vi "자판기.vi"() -> ()   [LabVIEW 2020]
panel:
  in  "정지":bool
  in  "거스름돈 반환":bool
  out "배출 상품명":string
  out "현재 잔액":dbl
  out "웰치스 LED":bool
  in  "웰치스":bool
  out "콜라 LED":bool
  in  "콜라":bool
  out "환타 LED":bool
  in  "환타":bool
  out "사이다 LED":bool
  in  "1000원":bool
  in  "500원":bool
  in  "100원":bool
  in  "10원":bool
  in  "50 원":bool
  in  "사이다":bool
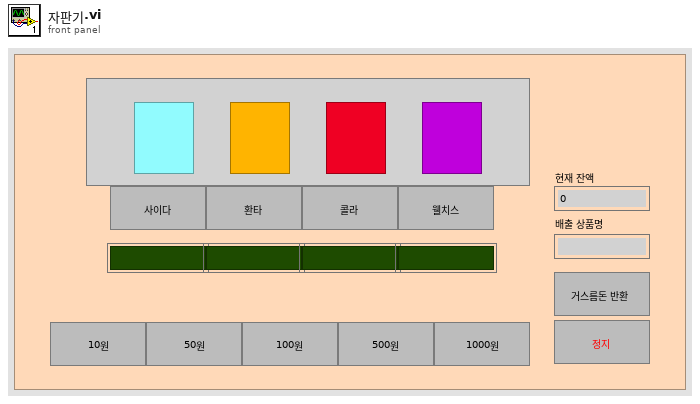
[diagram p1: front panel]
types:
  T1 = typedef "컨트롤 1.ctl" = enum16{"초기화", "대기", "10원", "50원", "100원", "500원", "1000원", "디스플레이 업데이트", "사이다", "콜라", "환타", "웰치스", "거스름돈 반환", "종료"}
  T2 = cluster{"배출 상품명":string, "현재 잔액":dbl, "웰치스 LED":bool, "콜라 LED":bool, "환타 LED":bool, "사이다 LED":bool}
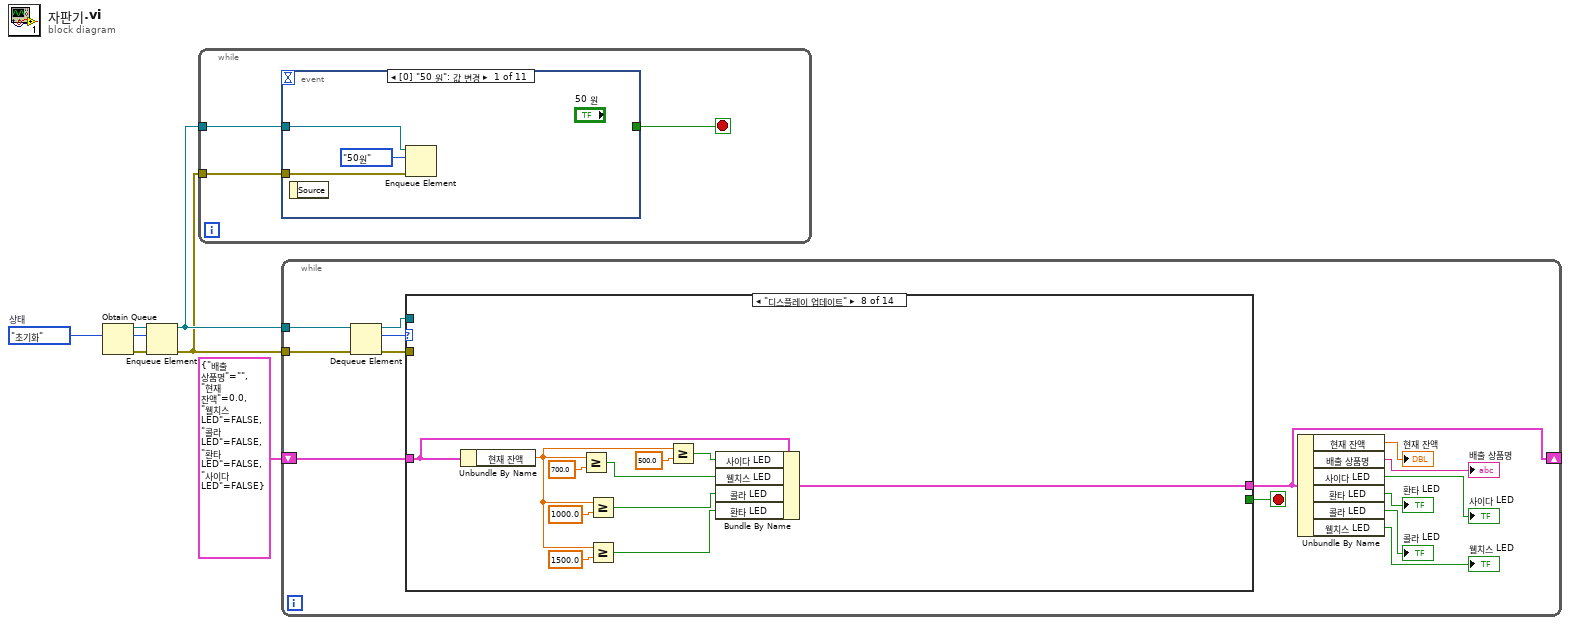
[diagram p0: block diagram]
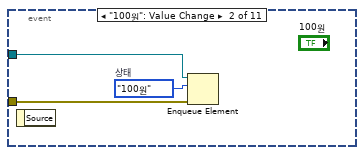
[diagram p2: hidden frame]
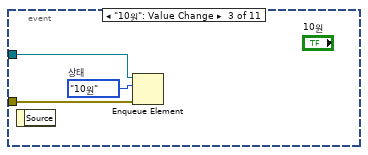
[diagram p3: hidden frame]
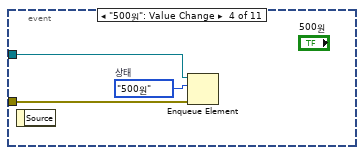
[diagram p4: hidden frame]
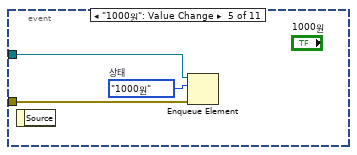
[diagram p5: hidden frame]
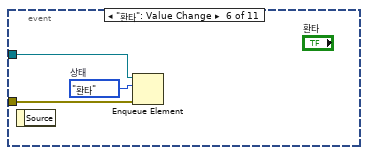
[diagram p6: hidden frame]
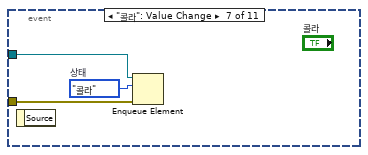
[diagram p7: hidden frame]
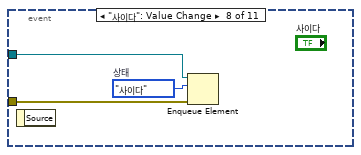
[diagram p8: hidden frame]
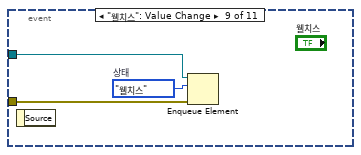
[diagram p9: hidden frame]
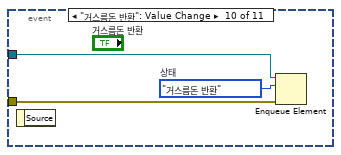
[diagram p10: hidden frame]
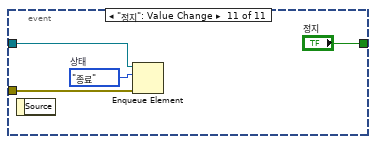
[diagram p11: hidden frame]
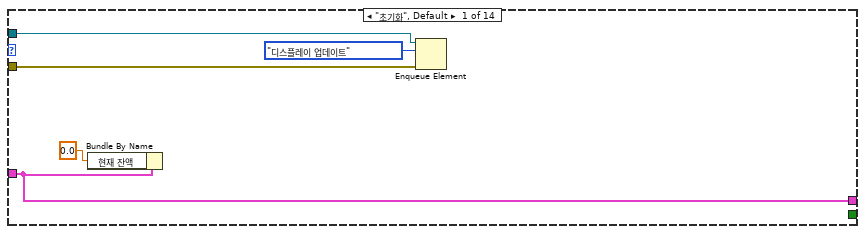
[diagram p12: hidden frame]
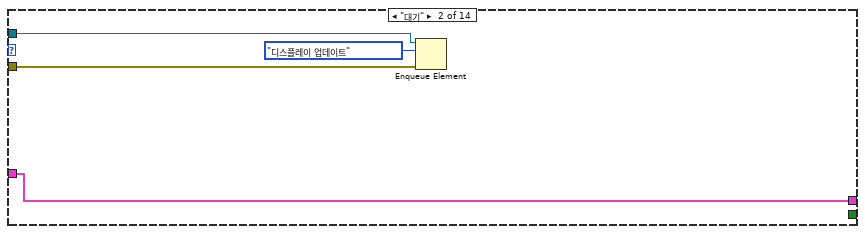
[diagram p13: hidden frame]
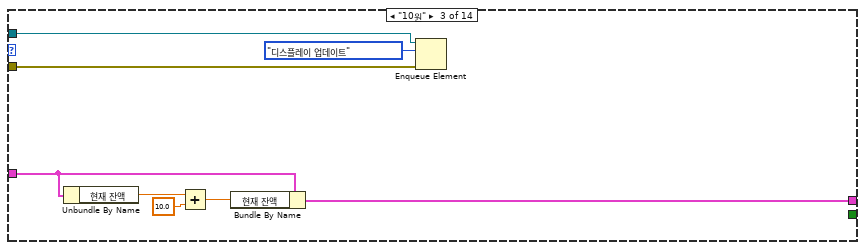
[diagram p14: hidden frame]
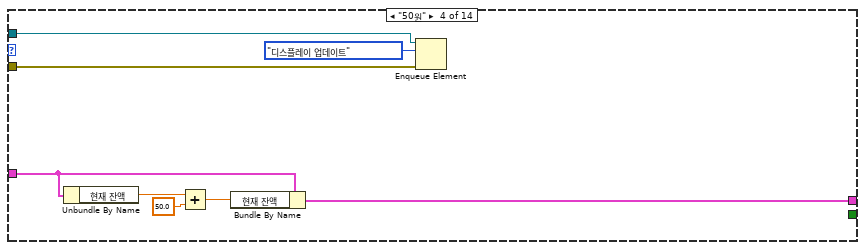
[diagram p15: hidden frame]
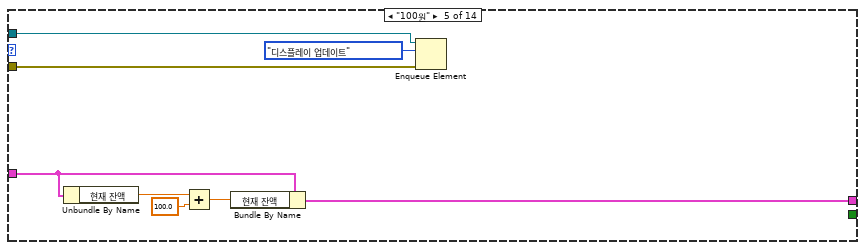
[diagram p16: hidden frame]
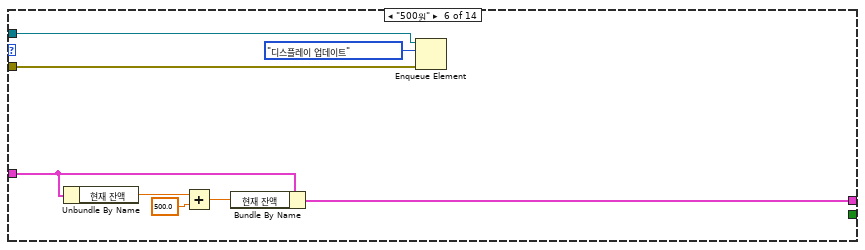
[diagram p17: hidden frame]
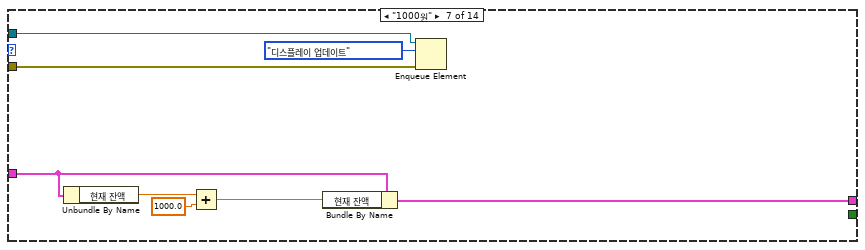
[diagram p18: hidden frame]
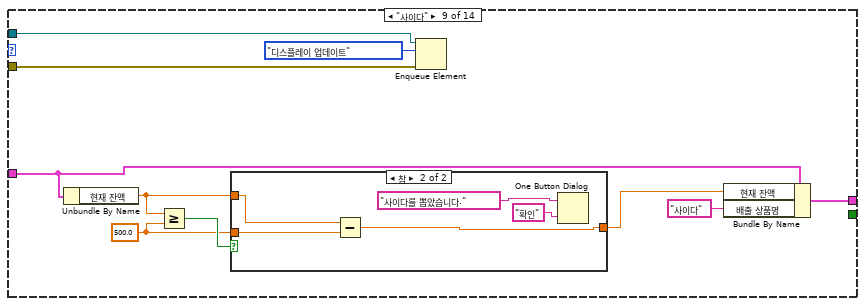
[diagram p19: hidden frame]
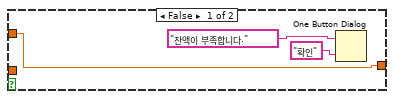
[diagram p20: hidden frame]
diagram:
  w4 = 컨트롤_1."초기화"  # 상태
  n1 = Obtain Queue(element data type=w4) -> (queue out=w5:refnum<queue>, error out=w3:errorcluster)  [unwired: 4 in, 1 out]
  n2 = Enqueue Element(queue=w5, element=w4, error in (no error)=w3) -> (queue out=w2:refnum<queue>, error out=w1:errorcluster)  [unwired: 1 in, 1 out]
  n3 = while {
    tunnel: w2 -> [w9]
    tunnel: w1 -> [w8]
    stop <- w7 stop-if-true
    n4 = event shown="[0] \"50 원\": 값 변경" {
      selector: _ -> [_ _ _ _ _ _ _ _ _ _ _]
      dyn-events: _ -> [_ _ _ _ _ _ _ _ _ _ _]
      timeout: _ -> [_ _ _ _ _ _ _ _ _ _ _]
      tunnel: w9 -> [w12 w15 w18 w21 w24 w27 w30 w33 w36 w39 w43]
      tunnel: w8 -> [w11 w14 w17 w20 w23 w26 w29 w32 w35 w38 w42]
      tunnel: [_ _ _ _ _ _ _ _ _ _ "정지"] -> w7
      event "50 원": Value Change {
        n5 = event-data() -> ()  [unwired: 1 in, 1 out]
        n6 = Enqueue Element(queue=w12, element=컨트롤_1."50원" ("원소"), error in (no error)=w11) -> ()  [unwired: 1 in, 3 out]
      }
      event "100원": Value Change {
        w13 = 컨트롤_1."100원"  # 상태
        n7 = event-data() -> ()  [unwired: 1 in, 1 out]
        n8 = Enqueue Element(queue=w15, element=w13, error in (no error)=w14) -> ()  [unwired: 1 in, 3 out]
      }
      event "10원": Value Change {
        w16 = 컨트롤_1."10원"  # 상태
        n9 = event-data() -> ()  [unwired: 1 in, 1 out]
        n10 = Enqueue Element(queue=w18, element=w16, error in (no error)=w17) -> ()  [unwired: 1 in, 3 out]
      }
      event "500원": Value Change {
        w19 = 컨트롤_1."500원"  # 상태
        n11 = event-data() -> ()  [unwired: 1 in, 1 out]
        n12 = Enqueue Element(queue=w21, element=w19, error in (no error)=w20) -> ()  [unwired: 1 in, 3 out]
      }
      event "1000원": Value Change {
        w22 = 컨트롤_1."1000원"  # 상태
        n13 = event-data() -> ()  [unwired: 1 in, 1 out]
        n14 = Enqueue Element(queue=w24, element=w22, error in (no error)=w23) -> ()  [unwired: 1 in, 3 out]
      }
      event "환타": Value Change {
        w25 = 컨트롤_1."환타"  # 상태
        n15 = event-data() -> ()  [unwired: 1 in, 1 out]
        n16 = Enqueue Element(queue=w27, element=w25, error in (no error)=w26) -> ()  [unwired: 1 in, 3 out]
      }
      event "콜라": Value Change {
        w28 = 컨트롤_1."콜라"  # 상태
        n17 = event-data() -> ()  [unwired: 1 in, 1 out]
        n18 = Enqueue Element(queue=w30, element=w28, error in (no error)=w29) -> ()  [unwired: 1 in, 3 out]
      }
      event "사이다": Value Change {
        w31 = 컨트롤_1."사이다"  # 상태
        n19 = event-data() -> ()  [unwired: 1 in, 1 out]
        n20 = Enqueue Element(queue=w33, element=w31, error in (no error)=w32) -> ()  [unwired: 1 in, 3 out]
      }
      event "웰치스": Value Change {
        w34 = 컨트롤_1."웰치스"  # 상태
        n21 = event-data() -> ()  [unwired: 1 in, 1 out]
        n22 = Enqueue Element(queue=w36, element=w34, error in (no error)=w35) -> ()  [unwired: 1 in, 3 out]
      }
      event "거스름돈 반환": Value Change {
        w37 = 컨트롤_1."거스름돈 반환"  # 상태
        n23 = event-data() -> ()  [unwired: 1 in, 1 out]
        n24 = Enqueue Element(queue=w39, element=w37, error in (no error)=w38) -> ()  [unwired: 1 in, 3 out]
      }
      event "정지": Value Change {
        w41 = 컨트롤_1."종료"  # 상태
        n25 = event-data() -> ()  [unwired: 1 in, 1 out]
        n26 = Enqueue Element(queue=w43, element=w41, error in (no error)=w42) -> ()  [unwired: 1 in, 3 out]
      }
    }
  }
  n27 = while {
    shift-right: [w56] -> _
    shift-left: T2 {"배출 상품명"="", "현재 잔액"=0.0, "웰치스 LED"=FALSE, "콜라 LED"=FALSE, "환타 LED"=FALSE, "사이다 LED"=FALSE} -> [w57]
    tunnel: w2 -> [w49]
    tunnel: w1 -> [w48]
    stop <- w44 stop-if-true
    n28 = Dequeue Element(queue=w49, error in (no error)=w48) -> (queue out=w46:refnum<queue>, element=w47:T1, error out=w45:errorcluster)  [unwired: 1 in, 1 out]
    n29 = case shown="\"디스플레이 업데이트\"" w47 {
      tunnel: w57 -> [w58 w63 w68 w80 w88 w92 w100 w113 w124 w141 w158 w177 w196 w202]
      tunnel: [w58 w63 w67 w78 w86 w91 w99 w107 w123 w140 w159 w174 w199 w202] -> w56
      tunnel: w46 -> [w61 w65 w70 w77 w85 w94 w102 _ w121 w139 w157 w176 w198 w204]
      tunnel: w45 -> [w60 w64 w69 w75 w83 w93 w101 _ w120 w138 w156 w175 w197 w203]
      tunnel: [_ _ _ _ _ _ _ _ _ _ _ _ _ TRUE] -> w44
      frame "초기화", Default {
        n30 = Bundle By Name(cluster=w58, "현재 잔액"=0.0) -> ()  [unwired: 1 out]
        n31 = Enqueue Element(queue=w61, element=컨트롤_1."디스플레이 업데이트" ("원소"), error in (no error)=w60) -> ()  [unwired: 1 in, 3 out]
      }
      frame "대기" {
        n32 = Enqueue Element(queue=w65, element=컨트롤_1."디스플레이 업데이트" ("원소"), error in (no error)=w64) -> ()  [unwired: 1 in, 3 out]
      }
      frame "10원" {
        n33 = Unbundle By Name(w68) -> ("현재 잔액"=w74:dbl)
        n34 = Add(x=w74, y=10.0) -> (x+y=w72:dbl)
        n35 = Bundle By Name(cluster=w68, "현재 잔액"=w72) -> (w67:T2)
        n36 = Enqueue Element(queue=w70, element=컨트롤_1."디스플레이 업데이트" ("원소"), error in (no error)=w69) -> ()  [unwired: 1 in, 3 out]
      }
      frame "50원" {
        n37 = Unbundle By Name(w80) -> ("현재 잔액"=w82:dbl)
        n38 = Add(x=w82, y=50.0) -> (x+y=w79:dbl)
        n39 = Bundle By Name(cluster=w80, "현재 잔액"=w79) -> (w78:T2)
        n40 = Enqueue Element(queue=w77, element=컨트롤_1."디스플레이 업데이트" ("원소"), error in (no error)=w75) -> ()  [unwired: 1 in, 3 out]
      }
      frame "100원" {
        n41 = Unbundle By Name(w88) -> ("현재 잔액"=w90:dbl)
        n42 = Add(x=w90, y=100.0) -> (x+y=w87:dbl)
        n43 = Bundle By Name(cluster=w88, "현재 잔액"=w87) -> (w86:T2)
        n44 = Enqueue Element(queue=w85, element=컨트롤_1."디스플레이 업데이트" ("원소"), error in (no error)=w83) -> ()  [unwired: 1 in, 3 out]
      }
      frame "500원" {
        n45 = Unbundle By Name(w92) -> ("현재 잔액"=w97:dbl)
        n46 = Add(x=w97, y=500.0) -> (x+y=w98:dbl)
        n47 = Bundle By Name(cluster=w92, "현재 잔액"=w98) -> (w91:T2)
        n48 = Enqueue Element(queue=w94, element=컨트롤_1."디스플레이 업데이트" ("원소"), error in (no error)=w93) -> ()  [unwired: 1 in, 3 out]
      }
      frame "1000원" {
        n49 = Unbundle By Name(w100) -> ("현재 잔액"=w105:dbl)
        n50 = Add(x=w105, y=1000.0) -> (x+y=w106:dbl)
        n51 = Bundle By Name(cluster=w100, "현재 잔액"=w106) -> (w99:T2)
        n52 = Enqueue Element(queue=w102, element=컨트롤_1."디스플레이 업데이트" ("원소"), error in (no error)=w101) -> ()  [unwired: 1 in, 3 out]
      }
      frame "디스플레이 업데이트" {
        n53 = Unbundle By Name(w113) -> ("현재 잔액"=w112:dbl)
        n54 = Greater Or Equal?(x=w112, y=700.0) -> (x >= y?=w110:bool)
        n55 = Greater Or Equal?(x=w112, y=1000.0) -> (x >= y?=w109:bool)
        n56 = Greater Or Equal?(x=w112, y=1500.0) -> (x >= y?=w108:bool)
        n57 = Greater Or Equal?(x=w112, y=500.0) -> (x >= y?=w111:bool)
        n58 = Bundle By Name(cluster=w113, "사이다 LED"=w111, "웰치스 LED"=w110, "콜라 LED"=w109, "환타 LED"=w108) -> (w107:T2)
      }
      frame "사이다" {
        w119 = 500.0 ("y")
        n59 = Unbundle By Name(w124) -> ("현재 잔액"=w126:dbl)
        n60 = Greater Or Equal?(x=w126, y=w119) -> (x >= y?=w127:bool)
        n61 = case shown="참" w127 {
          tunnel: w126 -> [w130 w135]
          tunnel: [w130 w134] -> w125
          tunnel: w119 -> [_ w131]
          frame False {
            n62 = One Button Dialog(message="잔액이 부족합니다." ("메시지"), button name ("OK")="확인" ("버튼 이름(\"확인\")")) -> ()  [unwired: 1 out]
          }
          frame True {
            n63 = Subtract(x=w135, y=w131) -> (x-y=w134:dbl)
            n64 = One Button Dialog(message="사이다를 뽑았습니다." ("메시지"), button name ("OK")="확인" ("버튼 이름(\"확인\")")) -> ()  [unwired: 1 out]
          }
        }
        n65 = Enqueue Element(queue=w121, element=컨트롤_1."디스플레이 업데이트" ("원소"), error in (no error)=w120) -> ()  [unwired: 1 in, 3 out]
        n66 = Bundle By Name(cluster=w124, "현재 잔액"=w125, "배출 상품명"="사이다") -> (w123:T2)
      }
      frame "콜라" {
        w137 = 1000.0 ("y")
        n67 = Unbundle By Name(w141) -> ("현재 잔액"=w144:dbl)
        n68 = Greater Or Equal?(x=w144, y=w137) -> (x >= y?=w145:bool)
        n69 = case shown="참" w145 {
          tunnel: w144 -> [w148 w153]
          tunnel: [w148 w152] -> w143
          tunnel: w137 -> [_ w149]
          frame False {
            n70 = One Button Dialog(message="잔액이 부족합니다." ("메시지"), button name ("OK")="확인" ("버튼 이름(\"확인\")")) -> ()  [unwired: 1 out]
          }
          frame True {
            n71 = Subtract(x=w153, y=w149) -> (x-y=w152:dbl)
            n72 = One Button Dialog(message="콜라를 뽑았습니다." ("메시지"), button name ("OK")="확인" ("버튼 이름(\"확인\")")) -> ()  [unwired: 1 out]
          }
        }
        n73 = Enqueue Element(queue=w139, element=컨트롤_1."디스플레이 업데이트" ("원소"), error in (no error)=w138) -> ()  [unwired: 1 in, 3 out]
        n74 = Bundle By Name(cluster=w141, "현재 잔액"=w143, "배출 상품명"="콜라") -> (w140:T2)
      }
      frame "환타" {
        w155 = 1500.0 ("y")
        n75 = Unbundle By Name(w158) -> ("현재 잔액"=w162:dbl)
        n76 = Greater Or Equal?(x=w162, y=w155) -> (x >= y?=w161:bool)
        n77 = case shown="참" w161 {
          tunnel: w162 -> [w166 w171]
          tunnel: [w166 w170] -> w163
          tunnel: w155 -> [_ w167]
          frame False {
            n78 = One Button Dialog(message="잔액이 부족합니다." ("메시지"), button name ("OK")="확인" ("버튼 이름(\"확인\")")) -> ()  [unwired: 1 out]
          }
          frame True {
            n79 = Subtract(x=w171, y=w167) -> (x-y=w170:dbl)
            n80 = One Button Dialog(message="환타를 뽑았습니다." ("메시지"), button name ("OK")="확인" ("버튼 이름(\"확인\")")) -> ()  [unwired: 1 out]
          }
        }
        n81 = Enqueue Element(queue=w157, element=컨트롤_1."디스플레이 업데이트" ("원소"), error in (no error)=w156) -> ()  [unwired: 1 in, 3 out]
        n82 = Bundle By Name(cluster=w158, "현재 잔액"=w163, "배출 상품명"="환타") -> (w159:T2)
      }
      frame "웰치스" {
        w173 = 700.0 ("y")
        n83 = Unbundle By Name(w177) -> ("현재 잔액"=w180:dbl)
        n84 = Greater Or Equal?(x=w180, y=w173) -> (x >= y?=w179:bool)
        n85 = case shown="참" w179 {
          tunnel: w180 -> [w184 w189]
          tunnel: [w184 w188] -> w181
          tunnel: w173 -> [_ w185]
          frame False {
            n86 = One Button Dialog(message="잔액이 부족합니다." ("메시지"), button name ("OK")="확인" ("버튼 이름(\"확인\")")) -> ()  [unwired: 1 out]
          }
          frame True {
            n87 = Subtract(x=w189, y=w185) -> (x-y=w188:dbl)
            n88 = One Button Dialog(message="웰치스를 뽑았습니다." ("메시지"), button name ("OK")="확인" ("버튼 이름(\"확인\")")) -> ()  [unwired: 1 out]
          }
        }
        n89 = Enqueue Element(queue=w176, element=컨트롤_1."디스플레이 업데이트" ("원소"), error in (no error)=w175) -> ()  [unwired: 1 in, 3 out]
        n90 = Bundle By Name(cluster=w177, "현재 잔액"=w181, "배출 상품명"="웰치스") -> (w174:T2)
      }
      frame "거스름돈 반환" {
        n91 = Unbundle By Name(w196) -> ("현재 잔액"=w194:dbl)
        n92 = Bundle By Name(cluster=w196, "현재 잔액"=0.0) -> (w199:T2)
        n93 = Number To Decimal String(number=w194) -> (decimal integer string=w193:string)  [unwired: 1 in]
        n94 = Concatenate Strings(w193, "원이 배출되었습니다." ("문자열")) -> (w191:string)
        n95 = Enqueue Element(queue=w198, element=컨트롤_1."디스플레이 업데이트" ("원소"), error in (no error)=w197) -> ()  [unwired: 1 in, 3 out]
        n96 = One Button Dialog(message=w191, button name ("OK")="확인" ("버튼 이름(\"확인\")")) -> ()  [unwired: 1 out]
      }
      frame "종료" {
        n97 = Enqueue Element(queue=w204, element=컨트롤_1."디스플레이 업데이트" ("원소"), error in (no error)=w203) -> ()  [unwired: 1 in, 3 out]
      }
    }
    n98 = Unbundle By Name(w56) -> ("현재 잔액"=→"현재 잔액":dbl, "배출 상품명"=→"배출 상품명":string, "사이다 LED"=→"사이다 LED":bool, "환타 LED"=→"환타 LED":bool, "콜라 LED"=→"콜라 LED":bool, "웰치스 LED"=→"웰치스 LED":bool)
  }
